vi "LSMcontroller_v64_updatedwaveformhandling.vi"() -> ()   [LabVIEW 2015] (continued)
                    n3086 = property on="wavdet" class="Bool (strict)"("Value"=FALSE ("wavdet")) -> ()  [unwired: 2 in, 2 out]
                    n3087 = local write "Save tab"(enum32{"withsave", "withoutsave"}."withsave" ("Save tab")) -> ()
                    n3088 = property on="# of frames" class="DigNum (strict)"("DisabledEnum"=T7."Enabled" ("Disabled")) -> ()  [unwired: 2 in, 2 out]
                    n3089 = property on="save\ndata" class="Bool (strict)"("DisabledEnum"=T7."Enabled" ("Disabled")) -> ()  [unwired: 2 in, 2 out]
                  }
                  frame True {
                    w6296 = FALSE ("finite samples for recording")
                    n3090 = property on="finite samples" class="Bool (strict)"("Value"=w6296) -> ()  [unwired: 2 in, 2 out]
                    n3091 = property on="wavdet" class="Bool (strict)"("Value"=w6296) -> ()  [unwired: 2 in, 2 out]
                    n3092 = property on="save\ndata" class="Bool (strict)"("Value"=w6296) -> ()  [unwired: 2 in, 2 out]
                    n3093 = local write "Save tab"(enum32{"withsave", "withoutsave"}."withsave" ("Save tab")) -> ()
                    n3094 = property on="# of frames" class="DigNum (strict)"("DisabledEnum"=T7."Disabled and Grayed Out" ("Disabled")) -> ()  [unwired: 2 in, 2 out]
                    n3095 = property on="save\ndata" class="Bool (strict)"("DisabledEnum"=T7."Disabled and Grayed Out" ("Disabled")) -> ()  [unwired: 2 in, 2 out]
                  }
                }
              }
              frame #1 {
                n3096 = local read "finite samples"() -> (w6306:bool)
                n3097 = local read "continuous"() -> (w6305:bool)
                n3098 = local read "wavdet"() -> (w6304:bool)
                n3099 = call "2pparameters.vi"("command"="get") -> ("params out"=w6300:T10)  [unwired: 1 in]
                n3100 = Bundle By Name(cluster=w6300, "finite"=w6306, "cont"=w6305, "wavdet"=w6304) -> (w6303:T10)
                n3101 = call "2pparameters.vi"("Params in"=w6303, "command"="set") -> ()  [unwired: 1 out]
              }
            }
          }
          event "wavdet": Value Change {
            n3102 = event-data() -> ("NewVal"=w6307:bool)  [unwired: 1 in]
            n3103 = flat-sequence {
              tunnel: w6307 -> [w6308]
              frame #0 {
                n3104 = case shown="False" w6308 {
                  frame False {
                    n3105 = property on="finite samples" class="Bool (strict)"("Value"=TRUE ("finite samples for recording")) -> ()  [unwired: 2 in, 2 out]
                    n3106 = property on="continuous" class="Bool (strict)"("Value"=FALSE ("continuous")) -> ()  [unwired: 2 in, 2 out]
                    n3107 = local write "Save tab"(enum32{"withsave", "withoutsave"}."withsave" ("Save tab")) -> ()
                    n3108 = property on="save\ndata" class="Bool (strict)"("DisabledEnum"=T7."Enabled" ("Disabled")) -> ()  [unwired: 2 in, 2 out]
                    n3109 = property on="# of frames" class="DigNum (strict)"("DisabledEnum"=T7."Enabled" ("Disabled")) -> ()  [unwired: 2 in, 2 out]
                    n3110 = property on="save\ndata" class="Bool (strict)"("Value"=TRUE ("save\ndata")) -> ()  [unwired: 2 in, 2 out]
                  }
                  frame True {
                    w6317 = FALSE ("finite samples for recording")
                    n3111 = property on="finite samples" class="Bool (strict)"("Value"=w6317) -> ()  [unwired: 2 in, 2 out]
                    n3112 = property on="continuous" class="Bool (strict)"("Value"=w6317) -> ()  [unwired: 2 in, 2 out]
                    n3113 = property on="save\ndata" class="Bool (strict)"("DisabledEnum"=T7."Enabled" ("Disabled")) -> ()  [unwired: 2 in, 2 out]
                    n3114 = local write "Save tab"(enum32{"withsave", "withoutsave"}."withsave" ("Save tab")) -> ()
                    n3115 = property on="# of frames" class="DigNum (strict)"("DisabledEnum"=T7."Disabled" ("Disabled")) -> ()  [unwired: 2 in, 2 out]
                    n3116 = property on="save\ndata" class="Bool (strict)"("Value"=TRUE ("save\ndata")) -> ()  [unwired: 2 in, 2 out]
                  }
                }
              }
              frame #1 {
                n3117 = local read "finite samples"() -> (w6320:bool)
                n3118 = local read "continuous"() -> (w6321:bool)
                n3119 = local read "wavdet"() -> (w6322:bool)
                n3120 = call "2pparameters.vi"("command"="get") -> ("params out"=w6326:T10)  [unwired: 1 in]
                n3121 = Bundle By Name(cluster=w6326, "finite"=w6320, "cont"=w6321, "wavdet"=w6322) -> (w6323:T10)
                n3122 = call "2pparameters.vi"("Params in"=w6323, "command"="set") -> ()  [unwired: 1 out]
              }
            }
          }
          event "cursors": Value Change {
            n3123 = event-data() -> ()  [unwired: 1 in, 5 out]
            n3124 = case shown="True" "cursors" {
              frame False {
                n3125 = property on="img_CH1" class="IntGraph (strict)"("Active Cursor"=u32 0, "Cursor.Cursor Style"=u8 0 ("Cursor Style"), "Cursor.Cursor Point Style"=u8 0 ("Cursor Point Style")) -> ("Cursor.Cursor Position:Cursor X"=w6331:dbl, "Cursor.Cursor Position:Cursor Y"=w6332:dbl)  [unwired: 2 in, 2 out]
                n3126 = property on="img_CH2" class="IntGraph (strict)"("Active Cursor"=u32 0, "Cursor.Cursor Style"=u8 0 ("Cursor Style"), "Cursor.Cursor Point Style"=u8 0 ("Cursor Point Style")) -> ()  [unwired: 2 in, 2 out]
                n3127 = local write "cursor x [pixel]"(w6331) -> ()
                n3128 = local write "cursor y [pixel]"(w6332) -> ()
              }
              frame True {
                n3129 = stacked-sequence {
                  frame #0 {
                    n3130 = call "2pparameters.vi"("command"="get") -> ("params out"=w6347:T10)  [unwired: 1 in]
                    n3131 = Unbundle By Name(w6347) -> ("Xpixels Img"=w6348:i32, "Ypixels Img"=w6345:i32)
                    n3132 = To Double Precision Float(number=w6345) -> (double precision float=w6339:dbl)
                    n3133 = To Double Precision Float(number=w6348) -> (double precision float=w6344:dbl)
                    n3134 = Divide(x=w6339, y=2.0) -> (x/y=w6340:dbl)
                    n3135 = Divide(x=w6344, y=2.0) -> (x/y=w6342:dbl)
                    n3136 = Round To Nearest(number=w6340) -> (nearest integer value=w6338:dbl)
                    n3137 = Round To Nearest(number=w6342) -> (nearest integer value=w6341:dbl)
                    n3138 = property on="img_CH1" class="IntGraph (strict)"("Active Cursor"=u32 0, "Cursor.Cursor Style"=u8 8 ("Cursor Style"), "Cursor.Cursor Point Style"=u8 5 ("Cursor Point Style"), "Cursor.Cursor Position:Cursor X"=w6341, "Cursor.Cursor Position:Cursor Y"=w6338, "Cursor.Visible"=TRUE) -> ()  [unwired: 2 in, 2 out]
                  }
                  frame #1 {
                    n3139 = call "2pparameters.vi"("command"="get") -> ("params out"=w6367:T10)  [unwired: 1 in]
                    n3140 = call "2pparameters.vi"("command"="get") -> ("params out"=w6365:T10)  [unwired: 1 in]
                    n3141 = property on="img_CH1" class="IntGraph (strict)"("Active Cursor"=u32 0, "Cursor.Cursor Style"=u8 8 ("Cursor Style"), "Cursor.Cursor Point Style"=u8 5 ("Cursor Point Style")) -> ("Cursor.Cursor Position:Cursor X"=w6360:dbl, "Cursor.Cursor Position:Cursor Y"=w6359:dbl, "Cursor.Cursor Index"=w6382:i32, "Cursor.Cursor Plot"=w6381:i32, "Cursor.Visible"=w6352:bool)  [unwired: 2 in, 2 out]
                    "cursor x [pixel]" <- w6360
                    "cursor y [pixel]" <- w6359
                    n3142 = Unbundle By Name(w6367) -> ("Vy-max Img"=w6369:dbl, "Vy-min Img"=w6356:dbl, "Ypixels Img"=w6371:i32)
                    n3143 = Unbundle By Name(w6365) -> ("VX-max Img"=w6366:dbl, "Vx-min Img"=w6354:dbl, "Xpixels Img"=w6370:i32)
                    n3144 = Subtract(x=w6369, y=w6356) -> (x-y=w6374:dbl)
                    n3145 = Subtract(x=w6366, y=w6354) -> (x-y=w6372:dbl)
                    n3146 = local read "img_CH2"() -> (w6378:sgl[][])
                    n3147 = To Double Precision Float(number=w6370) -> (double precision float=w6373:dbl)
                    n3148 = local read "img_CH1"() -> (w6379:sgl[][])
                    n3149 = To Double Precision Float(number=w6371) -> (double precision float=w6375:dbl)
                    n3150 = Index Array(array=w6379, index (row)=w6382, index (col)=w6381) -> (element=→"value CH 1":sgl)
                    n3151 = Index Array(array=w6378, index (row)=w6382, index (col)=w6381) -> (element=→"value CH 2":sgl)
                    n3152 = Divide(x=w6372, y=w6373) -> (x/y=w6376:dbl)
                    n3153 = Divide(x=w6374, y=w6375) -> (x/y=w6377:dbl)
                    n3154 = Multiply(x=w6360, y=w6376) -> (x*y=w6355:dbl)
                    n3155 = Multiply(x=w6359, y=w6377) -> (x*y=w6358:dbl)
                    n3156 = property on="img_CH2" class="IntGraph (strict)"("Active Cursor"=u32 0, "Cursor.Cursor Style"=u8 8 ("Cursor Style"), "Cursor.Cursor Point Style"=u8 5 ("Cursor Point Style"), "Cursor.Cursor Position:Cursor X"=w6360, "Cursor.Cursor Position:Cursor Y"=w6359, "Cursor.Visible"=w6352) -> ()  [unwired: 2 in, 2 out]
                    n3157 = Add(x=w6355, y=w6354) -> (x+y=w6353:dbl)
                    n3158 = Add(x=w6358, y=w6356) -> (x+y=w6357:dbl)
                    n3159 = local write "Vx-ref"(w6353) -> ()
                    n3160 = local write "Vy-ref"(w6357) -> ()
                  }
                }
              }
            }
          }
          event "img_CH1": Cursor Move {
            n3161 = event-data() -> ("CursIdx"=w6387:i32)  [unwired: 1 in]
            n3162 = Equal To 0?(x=w6387) -> (x = 0?=w6388:bool)
            n3163 = case shown="True" w6388 {
              frame False {
              }
              frame True {
                n3164 = call "2pparameters.vi"("command"="get") -> ("params out"=w6408:T10)  [unwired: 1 in]
                n3165 = call "2pparameters.vi"("command"="get") -> ("params out"=w6410:T10)  [unwired: 1 in]
                n3166 = property on="img_CH1" class="IntGraph (strict)"("Active Cursor"=u32 0, "Cursor.Cursor Style"=u8 8 ("Cursor Style"), "Cursor.Cursor Point Style"=u8 5 ("Cursor Point Style")) -> ("Cursor.Cursor Position:Cursor X"=w6397:dbl, "Cursor.Cursor Position:Cursor Y"=w6396:dbl, "Cursor.Cursor Plot"=w6416:i32, "Cursor.Cursor Index"=w6415:i32, "Cursor.Visible"=w6389:bool)  [unwired: 2 in, 2 out]
                n3167 = Unbundle By Name(w6408) -> ("Vy-max Img"=w6406:dbl, "Vy-min Img"=w6395:dbl, "Ypixels Img"=w6404:i32)
                n3168 = Unbundle By Name(w6410) -> ("VX-max Img"=w6409:dbl, "Vx-min Img"=w6390:dbl, "Xpixels Img"=w6405:i32)
                n3169 = Subtract(x=w6406, y=w6395) -> (x-y=w6401:dbl)
                n3170 = Subtract(x=w6409, y=w6390) -> (x-y=w6403:dbl)
                n3171 = local write "cursor x [pixel]"(w6397) -> ()
                n3172 = local write "cursor y [pixel]"(w6396) -> ()
                n3173 = To Double Precision Float(number=w6405) -> (double precision float=w6402:dbl)
                n3174 = To Double Precision Float(number=w6404) -> (double precision float=w6400:dbl)
                n3175 = local read "img_CH2"() -> (w6417:sgl[][])
                n3176 = local read "img_CH1"() -> (w6420:sgl[][])
                n3177 = Index Array(array=w6417, index (row)=w6416, index (col)=w6415) -> (element=w6418:sgl)
                n3178 = Index Array(array=w6420, index (row)=w6416, index (col)=w6415) -> (element=w6419:sgl)
                n3179 = Divide(x=w6403, y=w6402) -> (x/y=w6399:dbl)
                n3180 = Divide(x=w6401, y=w6400) -> (x/y=w6398:dbl)
                n3181 = local write "value CH 2"(w6418) -> ()
                n3182 = Multiply(x=w6397, y=w6399) -> (x*y=w6392:dbl)
                n3183 = local write "value CH 1"(w6419) -> ()
                n3184 = Multiply(x=w6396, y=w6398) -> (x*y=w6394:dbl)
                n3185 = Add(x=w6392, y=w6390) -> (x+y=w6391:dbl)
                n3186 = local write "Vx-ref"(w6391) -> ()
                n3187 = Add(x=w6394, y=w6395) -> (x+y=w6393:dbl)
                n3188 = property on="img_CH2" class="IntGraph (strict)"("Active Cursor"=u32 0, "Cursor.Cursor Style"=u8 8 ("Cursor Style"), "Cursor.Cursor Point Style"=u8 5 ("Cursor Point Style"), "Cursor.Cursor Position:Cursor X"=w6397, "Cursor.Cursor Position:Cursor Y"=w6396, "Cursor.Visible"=w6389) -> ()  [unwired: 2 in, 2 out]
                n3189 = local write "Vy-ref"(w6393) -> ()
              }
            }
          }
          event "img_CH2": Cursor Move {
            n3190 = event-data() -> ("CursIdx"=w6424:i32)  [unwired: 1 in]
            n3191 = Equal To 0?(x=w6424) -> (x = 0?=w6425:bool)
            n3192 = case shown="True" w6425 {
              frame False {
              }
              frame True {
                n3193 = property on="img_CH2" class="IntGraph (strict)"("Active Cursor"=u32 0, "Cursor.Cursor Style"=u8 8 ("Cursor Style"), "Cursor.Cursor Point Style"=u8 5 ("Cursor Point Style")) -> ("Cursor.Cursor Position:Cursor X"=w6433:dbl, "Cursor.Cursor Position:Cursor Y"=w6434:dbl, "Cursor.Cursor Plot"=w6453:i32, "Cursor.Cursor Index"=w6452:i32, "Cursor.Visible"=w6426:bool)  [unwired: 2 in, 2 out]
                n3194 = call "2pparameters.vi"("command"="get") -> ("params out"=w6445:T10)  [unwired: 1 in]
                n3195 = call "2pparameters.vi"("command"="get") -> ("params out"=w6447:T10)  [unwired: 1 in]
                n3196 = local read "img_CH1"() -> (w6457:sgl[][])
                n3197 = local read "img_CH2"() -> (w6454:sgl[][])
                n3198 = local write "cursor x [pixel]"(w6433) -> ()
                n3199 = local write "cursor y [pixel]"(w6434) -> ()
                n3200 = Unbundle By Name(w6445) -> ("Vy-max Img"=w6443:dbl, "Vy-min Img"=w6428:dbl, "Ypixels Img"=w6441:i32)
                n3201 = Unbundle By Name(w6447) -> ("VX-max Img"=w6446:dbl, "Vx-min Img"=w6431:dbl, "Xpixels Img"=w6442:i32)
                n3202 = Index Array(array=w6457, index (row)=w6453, index (col)=w6452) -> (element=w6456:sgl)
                n3203 = Index Array(array=w6454, index (row)=w6453, index (col)=w6452) -> (element=w6455:sgl)
                n3204 = local write "value CH 2"(w6455) -> ()
                n3205 = local write "value CH 1"(w6456) -> ()
                n3206 = Subtract(x=w6443, y=w6428) -> (x-y=w6438:dbl)
                n3207 = Subtract(x=w6446, y=w6431) -> (x-y=w6440:dbl)
                n3208 = To Double Precision Float(number=w6442) -> (double precision float=w6439:dbl)
                n3209 = To Double Precision Float(number=w6441) -> (double precision float=w6437:dbl)
                n3210 = Divide(x=w6440, y=w6439) -> (x/y=w6436:dbl)
                n3211 = Divide(x=w6438, y=w6437) -> (x/y=w6435:dbl)
                n3212 = Multiply(x=w6433, y=w6436) -> (x*y=w6432:dbl)
                n3213 = Multiply(x=w6434, y=w6435) -> (x*y=w6429:dbl)
                n3214 = property on="img_CH1" class="IntGraph (strict)"("Active Cursor"=u32 0, "Cursor.Cursor Style"=u8 8 ("Cursor Style"), "Cursor.Cursor Point Style"=u8 5 ("Cursor Point Style"), "Cursor.Cursor Position:Cursor X"=w6433, "Cursor.Cursor Position:Cursor Y"=w6434, "Cursor.Visible"=w6426) -> ()  [unwired: 2 in, 2 out]
                n3215 = Add(x=w6432, y=w6431) -> (x+y=→"Vx-ref":dbl)
                n3216 = Add(x=w6429, y=w6428) -> (x+y=→"Vy-ref":dbl)
              }
            }
          }
          event "Focus": Value Change {
            n3217 = event-data() -> ()  [unwired: 1 in, 6 out]
            n3218 = flat-sequence {
              frame #0 {
                n3219 = local read "Focus"() -> (w6461:bool)
                n3220 = case shown="True" w6461 {
                  frame False {
                  }
                  frame True {
                    n3221 = local read "Vx-ref"() -> (w6465:dbl)
                    n3222 = local read "Vy-ref"() -> (w6464:dbl)
                    n3223 = local read "zV"() -> (w6462:dbl)
                    n3224 = call "focusvi.vi"("zc"=w6462, "yc"=w6464, "xc"=w6465) -> ("finalz"=→"zV":dbl)
                  }
                }
              }
              frame #1 {
                n3225 = local write "Focus"(FALSE ("Focus")) -> ()
              }
            }
          }
          event "auto shutter": Value Change {
            n3226 = event-data() -> ()  [unwired: 1 in, 6 out]
            n3227 = call "2pparameters.vi"("command"="get") -> ("params out"=w6469:T10)  [unwired: 1 in]
            n3228 = in-place {
              n3229 = in-place-cluster #46(w6469) -> ()  [unwired: 1 out]
              n3230 = local read "auto shutter"() -> (w6471:bool)
              n3231 = in-place-cluster #46("autoshutter"=w6471) -> (w6467:T10)
            }
            n3232 = call "2pparameters.vi"("Params in"=w6467, "command"="set") -> ()  [unwired: 1 out]
          }
          event "auto OD": Value Change {
            n3233 = event-data() -> ()  [unwired: 1 in, 6 out]
            n3234 = call "2pparameters.vi"("command"="get") -> ("params out"=w6474:T10)  [unwired: 1 in]
            n3235 = in-place {
              n3236 = in-place-cluster #47(w6474) -> ()  [unwired: 1 out]
              n3237 = local read "auto OD"() -> (w6476:bool)
              n3238 = in-place-cluster #47("auto OD"=w6476) -> (w6472:T10)
            }
            n3239 = call "2pparameters.vi"("Params in"=w6472, "command"="set") -> ()  [unwired: 1 out]
          }
          event "ODfilt": Value Change {
            n3240 = event-data() -> ("OldVal"=w6477:u16)  [unwired: 1 in, 5 out]
            n3241 = local read "ODfilt"() -> (w6478:u16)
            n3242 = call "2pparameters.vi"("command"="get") -> ("params out"=w6481:T10)  [unwired: 1 in]
            n3243 = call "filterwheelcontrol_nothorlabslib.vi"("Current OD filt"=w6477, "New ODfilt"=w6478) -> ()  [unwired: 1 in]
            n3244 = in-place {
              in-place-border: w6478 -> [w6483]
              n3245 = in-place-cluster #48(w6481) -> ()  [unwired: 1 out]
              n3246 = in-place-cluster #48("ODfilt"=w6483) -> (w6479:T10)
            }
            n3247 = call "2pparameters.vi"("Params in"=w6479, "command"="set") -> ()  [unwired: 1 out]
          }
          event "Exit": Value Change {
            n3248 = event-data() -> ()  [unwired: 1 in, 5 out]
          }
        }
        n3249 = Wait (ms)(milliseconds to wait=u32 50) -> ()  [unwired: 1 out]
      }
      n3250 = while {
        stop <- w69 stop-if-true
        # "Waveform generation"
        n3251 = event shown="[15] \"Update settings\": Value Change" {
          selector: _ -> [_ _ _ _ _ _ _ _ _ _ _ _ _ _ _ _ _ _ _ _ _ _]
          dyn-events: _ -> [_ _ _ _ _ _ _ _ _ _ _ _ _ _ _ _ _ _ _ _ _ _]
          timeout: _ -> [_ _ _ _ _ _ _ _ _ _ _ _ _ _ _ _ _ _ _ _ _ _]
          tunnel: [_ _ _ _ _ _ _ _ _ _ _ _ _ _ _ _ _ _ _ _ _ w2081] -> w69
          event Timeout {
            n3252 = event-data() -> ()  [unwired: 1 in, 3 out]
          }
          event "Add AO wave": Value Change {
            n3253 = event-data() -> ("NewVal"=w70:bool)  [unwired: 1 in, 5 out]
            n3254 = case shown="True" w70 {
              frame False {
              }
              frame True {
                n3255 = stacked-sequence {
                  frame #0 {
                    n3256 = local read "Measurement"() -> (w71:T4)
                    n3257 = case shown="\"Lifetime (contour)\"" w71 {
                      frame "X-Y-t movie", Default {
                        n3258 = local read "avpp"() -> (w92:i32)
                        n3259 = local read "Angle ref"() -> (w91:dbl)
                        n3260 = local read "ROI Type"() -> (w90:u16)
                        n3261 = local read "xpixels ref"() -> (w87:i32)
                        n3262 = local read "Vx-min ref"() -> (w86:dbl)
                        n3263 = local read "Vx-max ref"() -> (w85:dbl)
                        n3264 = local read "ypixels ref"() -> (w83:i32)
                        n3265 = local read "Vy-min ref"() -> (w84:dbl)
                        n3266 = local read "Vy-max ref"() -> (w80:dbl)
                        n3267 = local read "Sampling rate"() -> (w74:dbl)
                        n3268 = local read "finite samples"() -> (w75:bool)
                        n3269 = local read "continuous"() -> (w78:bool)
                        n3270 = local read "wavdet"() -> (w79:bool)
                        n3271 = local read "# of frames"() -> (w77:i32)
                        n3272 = local read "maxbufferAI"() -> (w76:i32)
                        n3273 = local read "Override AI buffer"() -> (w72:bool)
                        n3274 = call "2pparameters.vi"("command"="get") -> ("params out"=w89:T10)  [unwired: 1 in]
                        n3275 = Bundle By Name(cluster=w89, "type"="X-Y-t movie", "avpp"=w92, "Angle Img"=w91, "Xpixels Img"=w87, "Vx-min Img"=w86, "VX-max Img"=w85, "Ypixels Img"=w83, "Vy-min Img"=w84, "Vy-max Img"=w80, "srate"=w74, "srate Img"=w74, "finite"=w75, "cont"=w78, "wavdet"=w79, "measpoints"=w77, "maxbufferAI"=w76, "Drawing Mode"=w90, "Vz-reset"=0.0, "AIoverride"=w72) -> (w81:T10)
                        n3276 = call "2pparameters.vi"("Params in"=w81, "command"="set") -> ()  [unwired: 1 out]
                      }
                      frame "X-Y-Z stack" {
                        n3277 = call "2pparameters.vi"("command"="get") -> ("params out"=w96:T10)  [unwired: 1 in]
                        n3278 = Bundle By Name(cluster=w96, "type"="X-Y-Z stack") -> (w94:T10)
                        n3279 = call "2pparameters.vi"("Params in"=w94, "command"="set") -> ()  [unwired: 1 out]
                      }
                      frame "Lifetime (scan)" {
                        n3280 = call "2pparameters.vi"("command"="get") -> ("params out"=w101:T10)  [unwired: 1 in]
                        n3281 = Bundle By Name(cluster=w101, "type"="Lifetime (scan)") -> (w99:T10)
                        n3282 = call "2pparameters.vi"("Params in"=w99, "command"="set") -> ()  [unwired: 1 out]
                      }
                      frame "Lifetime (contour)" {
                        n3283 = local read "Vy-min draw"() -> (w111:dbl)
                        n3284 = local read "Vy-max draw"() -> (w110:dbl)
                        n3285 = local read "Vx-min draw"() -> (w113:dbl)
                        n3286 = local read "Vx-max draw"() -> (w112:dbl)
                        n3287 = local read "xpixels ref"() -> (w109:i32)
                        n3288 = local read "ypixels ref"() -> (w108:i32)
                        n3289 = local read "ROI Type"() -> (w107:u16)
                        n3290 = local read "srateAODOtt"() -> (w118:dbl)
                        n3291 = local read "# of frames"() -> (w123:i32)
                        n3292 = local read "refreshtime"() -> (w115:dbl)
                        n3293 = local read "Pel"() -> (w106:dbl)
                        n3294 = local read "bin"() -> (w121:dbl)
                        n3295 = local read "Override AI buffer"() -> (w104:bool)
                        n3296 = local read "finite samples"() -> (w130:bool)
                        n3297 = local read "srateAODOtt"() -> (w117:dbl)
                        n3298 = local read "srateAODOtt"() -> (w124:dbl)
                        n3299 = local read "continuous"() -> (w129:bool)
                        n3300 = local read "Angle ref"() -> (w114:dbl)
                        n3301 = local read "wavdet"() -> (w131:bool)
                        n3302 = local read "Vx-ref"() -> (w126:dbl)
                        n3303 = local read "Vy-ref"() -> (w128:dbl)
                        n3304 = local read "avpp"() -> (w127:i32)
                        n3305 = call "tt_timeandsamples.vi"("bin"=w121, "refreshtime"=w115, "srateAODOtt"=w118, "tot#ofsamples"=w123) -> ("refreshrate"=w119:dbl, "refreshbuffer"=w120:i32, "timetracecycles"=w125:i32)  [unwired: 5 in]
                        n3306 = local read "bin"() -> (w122:dbl)
                        n3307 = call "2pparameters.vi"("command"="get") -> ("params out"=w134:T10)  [unwired: 1 in]
                        n3308 = Bundle By Name(cluster=w134, "Drawing Mode"=w107, "measpoints"=w123, "tt_cycles"=w125, "refreshbuffer"=w120, "refreshrate"=w119, "Vx-ref"=w126, "Vy-ref"=w128, "srate"=w117, "finite"=w130, "cont"=w129, "wavdet"=w131, "avpp"=w127, "srateAODO"=w124, "bufferAI"=w120, "bin"=w122, "Angle Img"=w114, "Vxminref"=w113, "Vxmaxref"=w112, "Vyminref"=w111, "Vymaxref"=w110, "Xpixels Img"=w109, "Ypixels Img"=w108, "Pel"=w106, "Vz-reset"=0.0, "AIoverride"=w104, "type"="Lifetime (contour)") -> (w132:T10)
                        n3309 = Reciprocal(x=w119) -> (1/x=w116:dbl)
                        n3310 = local write "refreshtime"(w116) -> ()
                        n3311 = call "2pparameters.vi"("Params in"=w132, "command"="set") -> ()  [unwired: 1 out]
                      }
                      frame "X-Y-Z-t movie" {
                      }
                      frame "linescan" {
                      }
                      frame "Timetrace" {
                        n3312 = local read "Vy-min draw"() -> (w144:dbl)
                        n3313 = local read "Vy-max draw"() -> (w143:dbl)
                        n3314 = local read "Vx-min draw"() -> (w146:dbl)
                        n3315 = local read "Vx-max draw"() -> (w145:dbl)
                        n3316 = local read "xpixels ref"() -> (w142:i32)
                        n3317 = local read "ypixels ref"() -> (w141:i32)
                        n3318 = local read "ROI Type"() -> (w140:u16)
                        n3319 = local read "srateAODOtt"() -> (w151:dbl)
                        n3320 = local read "# of frames"() -> (w156:i32)
                        n3321 = local read "refreshtime"() -> (w148:dbl)
                        n3322 = local read "Pel"() -> (w139:dbl)
                        n3323 = local read "bin"() -> (w154:dbl)
                        n3324 = local read "Override AI buffer"() -> (w137:bool)
                        n3325 = local read "finite samples"() -> (w163:bool)
                        n3326 = local read "srateAODOtt"() -> (w150:dbl)
                        n3327 = local read "srateAODOtt"() -> (w157:dbl)
                        n3328 = local read "continuous"() -> (w162:bool)
                        n3329 = local read "Angle ref"() -> (w147:dbl)
                        n3330 = local read "wavdet"() -> (w164:bool)
                        n3331 = local read "Vx-ref"() -> (w159:dbl)
                        n3332 = local read "Vy-ref"() -> (w161:dbl)
                        n3333 = local read "avpp"() -> (w160:i32)
                        n3334 = call "tt_timeandsamples.vi"("bin"=w154, "refreshtime"=w148, "srateAODOtt"=w151, "tot#ofsamples"=w156) -> ("refreshrate"=w152:dbl, "refreshbuffer"=w153:i32, "timetracecycles"=w158:i32)  [unwired: 5 in]
                        n3335 = local read "bin"() -> (w155:dbl)
                        n3336 = call "2pparameters.vi"("command"="get") -> ("params out"=w167:T10)  [unwired: 1 in]
                        n3337 = Bundle By Name(cluster=w167, "Drawing Mode"=w140, "measpoints"=w156, "tt_cycles"=w158, "refreshbuffer"=w153, "refreshrate"=w152, "Vx-ref"=w159, "Vy-ref"=w161, "srate"=w150, "finite"=w163, "cont"=w162, "wavdet"=w164, "avpp"=w160, "srateAODO"=w157, "bufferAI"=w153, "bin"=w155, "Angle Img"=w147, "Vxminref"=w146, "Vxmaxref"=w145, "Vyminref"=w144, "Vymaxref"=w143, "Xpixels Img"=w142, "Ypixels Img"=w141, "Pel"=w139, "Vz-reset"=0.0, "AIoverride"=w137, "type"="Timetrace") -> (w165:T10)
                        n3338 = Reciprocal(x=w152) -> (1/x=w149:dbl)
                        n3339 = local write "refreshtime"(w149) -> ()
                        n3340 = call "2pparameters.vi"("Params in"=w165, "command"="set") -> ()  [unwired: 1 out]
                      }
                      frame "Lifetime (point)" {
                      }
                    }
                  }
                  frame #1 {
                    w170 = FALSE ("wavdet")
                    n3341 = call "2pparameters.vi"("command"="get") -> ("params out"=w174:T10)  [unwired: 1 in]
                    n3342 = Bundle By Name(cluster=w174, "finite"=w170, "cont"=w170, "wavdet"=TRUE) -> (w171:T10)
                    n3343 = call "2pparameters.vi"("Params in"=w171, "command"="set") -> ()  [unwired: 1 out]
                  }
                  frame #2 {
                    # "change active waveform numbers array"
                    n3344 = local read "AO channels"() -> (w181:u32)
                    n3345 = call "2pparameters.vi"("command"="get") -> ("params out"=w179:T10)  [unwired: 1 in]
                    n3346 = in-place {
                      in-place-border: w181 -> [w185]
                      in-place-border: [w182] -> w176
                      n3347 = in-place-cluster #49(w179) -> ("aAO"=w184:u32[])
                      n3348 = call "add channel to active arrayv2.vi"("line array in"=w184, "line to add"=w185) -> ("line array out"=w183:u32[], "addition"=w182:bool)  [unwired: 1 out]
                      n3349 = in-place-cluster #49("aAO"=w183) -> (w177:T10)
                    }
                    n3350 = local write "addAO"(w176) -> ()
                    n3351 = call "2pparameters.vi"("Params in"=w177, "command"="set") -> ()  [unwired: 1 out]
                  }
                  frame #3 {
                    # "update GUI"
                    n3352 = local read "addAO"() -> (w186:bool)
                    n3353 = case shown="True" w186 {
                      frame False {
                      }
                      frame True {
                        n3354 = call "Used AO lines.vi"() -> ("used AO names"=w190:string[], "used AO lines"=w192:tag[])  [unwired: 2 in]
                        n3355 = control-ref of="Analog Lines Plot"() -> (w191:refnum<vi>)
                        n3356 = control-ref of="Digital Lines Plot"() -> (w189:refnum<vi>)
                        n3357 = call "Used DO lines.vi"() -> ("used DO names"=w188:string[], "used DO lines"=w187:tag[])  [unwired: 2 in]
                        n3358 = local write "Analog Used Lines"(w192) -> ()
                        n3359 = local write "Analog Used Names"(w190) -> ()
                        n3360 = local write "Digital Used Lines"(w187) -> ()
                        n3361 = local write "Digital Used Names"(w188) -> ()
                        n3362 = call "prepDOWaveplot.vi"("DigitalGraph in"=w189, "used DO names"=w188) -> ()  [unwired: 1 in]
                        n3363 = call "prepAOWaveplot.vi"("WaveformGraph in"=w191, "Analog Used Names"=w190) -> ()  [unwired: 1 in]
                      }
                    }
                  }
                  frame #4 {
                    n3364 = local read "addAO"() -> (w193:bool)
                    n3365 = case shown="True" w193 {
                      frame False {
                      }
                      frame True {
                        # "add parameters\nto parameter array"
                        n3366 = local read "Build analog waveform tabs"() -> (w194:enum32{"Square", "Triangle", "Matlab"})
                        n3367 = case shown="\"Matlab\"" w194 {
                          frame "Square", Default {
                            w207 = 0.0 ("Offset (V)")
                            n3368 = local read "Meastab"() -> (w196:enum32{"X-Y Image", "Linescan", "Timetrace"})
                            n3369 = call "waveformparamsv2.vi"("command"="get") -> ("Params out"=w205:T14)  [unwired: 4 in, 2 out]
                            n3370 = Unbundle By Name(w205) -> ("AO parameters"=w202:T15)
                            n3371 = case shown="\"Timetrace\"" w196 {
                              tunnel: [w218 w219] -> w195
                              frame "X-Y Image", Default {
                                n3372 = local read "Sampling rate"() -> (w218:dbl)
                              }
                              frame "Timetrace" {
                                n3373 = local read "srateAODOtt"() -> (w219:dbl)
                              }
                            }
                            n3374 = local read "Start amplitude (V)"() -> (w215:dbl)
                            n3375 = local read "phase shift (ms)"() -> (w208:dbl)
                            n3376 = local read "Step size (V)"() -> (w213:dbl)
                            n3377 = local read "Baseline (V)"() -> (w214:dbl)
                            n3378 = local read "Period (ms)"() -> (w211:dbl)
                            n3379 = local read "padding value"() -> (w198:dbl)
                            n3380 = local read "Repeats"() -> (w217:dbl)
                            n3381 = local read "DC (%)"() -> (w212:dbl)
                            n3382 = local read "Cycles"() -> (w216:dbl)
                            n3383 = local read "Pulses"() -> (w209:dbl)
                            n3384 = Index Array(array=w202, index=0) -> (element=w203:T16)
                            n3385 = Bundle By Name(cluster=w203, "AOtab"=0.0 ("Repeats"), "Repeats"=w217, "Cycles"=w216, "Start amplitude (V)"=w215, "Baseline (V)"=w214, "Step size (V)"=w213, "DC (%)"=w212, "Sampling frequency (Hz)"=w195, "Period (ms)"=w211, "Offset (V)"=w207, "Amplitude (V)"=w207, "Frequency"=w207, "Tri Repeats"=w207, "phase shift (ms)"=w208, "Pulses"=w209, "Matlab wave file"=path "", "padding value"=w198) -> (w200:T16)
                            n3386 = Build Array(w200) -> (w199:T15)
                            n3387 = call "waveformparamsv2.vi"("command"="add AO", "add AO"=w199) -> ()  [unwired: 3 in, 3 out]
                          }
                          frame "Matlab" {
                            w225 = 0.0 ("Repeats")
                            n3388 = local read "Meastab"() -> (w221:enum32{"X-Y Image", "Linescan", "Timetrace"})
                            n3389 = call "waveformparamsv2.vi"("command"="get") -> ("Params out"=w232:T14)  [unwired: 4 in, 2 out]
                            n3390 = Unbundle By Name(w232) -> ("AO parameters"=w229:T15)
                            n3391 = case shown="\"Timetrace\"" w221 {
                              tunnel: [w235 w236] -> w220
                              frame "X-Y Image", Default {
                                n3392 = local read "Sampling rate"() -> (w235:dbl)
                              }
                              frame "Timetrace" {
                                n3393 = local read "srateAODOtt"() -> (w236:dbl)
                              }
                            }
                            n3394 = local read "Matlab waveform path"() -> (w222:path)
                            n3395 = local read "Matlab padding value"() -> (w224:dbl)
                            n3396 = Index Array(array=w229, index=0) -> (element=w230:T16)
                            n3397 = call "matlabwfexistsdialogue.vi"("Matlab waveform path"=w222) -> ("mtalab waveform path out"=w223:path)
                            n3398 = Bundle By Name(cluster=w230, "AOtab"=2.0 ("Repeats"), "Repeats"=w225, "Cycles"=w225, "Start amplitude (V)"=w225, "Baseline (V)"=w225, "Step size (V)"=w225, "DC (%)"=w225, "Sampling frequency (Hz)"=w220, "Period (ms)"=w225, "Offset (V)"=w225, "Amplitude (V)"=w225, "Frequency"=w225, "Tri Repeats"=w225, "phase shift (ms)"=w225, "Pulses"=w225, "Matlab wave file"=w223, "padding value"=w224) -> (w227:T16)
                            n3399 = Build Array(w227) -> (w226:T15)
                            n3400 = call "waveformparamsv2.vi"("command"="add AO", "add AO"=w226) -> ()  [unwired: 3 in, 3 out]
                          }
                          frame "Triangle" {
                            w242 = 0.0 ("Offset (V)")
                            n3401 = local read "Meastab"() -> (w238:enum32{"X-Y Image", "Linescan", "Timetrace"})
                            n3402 = call "waveformparamsv2.vi"("command"="get") -> ("Params out"=w254:T14)  [unwired: 4 in, 2 out]
                            n3403 = Unbundle By Name(w254) -> ("AO parameters"=w251:T15)
                            n3404 = case shown="\"Timetrace\"" w238 {
                              tunnel: [w256 w257] -> w237
                              frame "X-Y Image", Default {
                                n3405 = local read "Sampling rate"() -> (w256:dbl)
                              }
                              frame "Timetrace" {
                                n3406 = local read "srateAODOtt"() -> (w257:dbl)
                              }
                            }
                            n3407 = local read "Tri padding value"() -> (w240:dbl)
                            n3408 = local read "Amplitude (V)"() -> (w245:dbl)
                            n3409 = local read "Tri Phase (s)"() -> (w241:dbl)
                            n3410 = local read "Tri Repeats"() -> (w243:dbl)
                            n3411 = local read "Frequency"() -> (w244:dbl)
                            n3412 = local read "Offset (V)"() -> (w246:dbl)
                            n3413 = Index Array(array=w251, index=0) -> (element=w252:T16)
                            n3414 = Bundle By Name(cluster=w252, "AOtab"=1.0 ("Repeats"), "Repeats"=w242, "Cycles"=w242, "Start amplitude (V)"=w242, "Baseline (V)"=w242, "Step size (V)"=w242, "DC (%)"=w242, "Sampling frequency (Hz)"=w237, "Period (ms)"=w242, "Offset (V)"=w246, "Amplitude (V)"=w245, "Frequency"=w244, "Tri Repeats"=w243, "phase shift (ms)"=w242, "Pulses"=w242, "Matlab wave file"=path "", "Tri phase"=w241, "padding value"=w240) -> (w249:T16)
                            n3415 = Build Array(w249) -> (w248:T15)
                            n3416 = call "waveformparamsv2.vi"("command"="add AO", "add AO"=w248) -> ()  [unwired: 3 in, 3 out]
                          }
                        }
                      }
                    }
                  }
                  frame #5 {
                    n3417 = local read "addAO"() -> (w258:bool)
                    n3418 = case shown="True" w258 {
                      frame False {
                      }
                      frame True {
                        # "add waveform to waveform array; correct waveform lengths and plot"
                        n3419 = local read "Meastab"() -> (w262:enum32{"X-Y Image", "Linescan", "Timetrace"})
                        n3420 = local read "Build analog waveform tabs"() -> (w272:enum32{"Square", "Triangle", "Matlab"})
                        n3421 = case shown="\"Timetrace\"" w262 {
                          tunnel: [w280 w281] -> w261
                          frame "X-Y Image", Default {
                            n3422 = local read "Sampling rate"() -> (w280:dbl)
                          }
                          frame "Timetrace" {
                            n3423 = local read "srateAODOtt"() -> (w281:dbl)
                          }
                        }
                        n3424 = call "waveformparamsv2.vi"("command"="get last AO") -> ("last AO"=w274:T16)  [unwired: 4 in, 2 out]
                        n3425 = case shown="\"Matlab\"" w272 {
                          tunnel: w274 -> [w284 w286 w288]
                          tunnel: [w283 w285 w287] -> w273
                          frame "Square", Default {
                            n3426 = call "generateRampedSquareWave_fromAOparameters.vi"("AO params"=w284) -> ("Waveform"=w283:waveform(dbl))  [unwired: 1 out]
                          }
                          frame "Triangle" {
                            n3427 = call "generateTriWave_fromAOparameters.vi"("AO params"=w286) -> ("Waveform"=w285:waveform(dbl))  [unwired: 1 out]
                          }
                          frame "Matlab" {
                            n3428 = call "matlabAOwffromparam.vi"("Cluster"=w288) -> ("Waveform"=w287:waveform(dbl))  [unwired: 1 out]
                          }
                        }
                        n3429 = property on="refwf" class="Ring (strict)"() -> ("RingText.Text"=w265:string)  [unwired: 2 in, 2 out]
                        n3430 = call "waveformsAObuffer.vi"("command"="get") -> ("AO wf out"=w278:waveform(dbl)[])  [unwired: 1 in]
                        n3431 = Build Array (concatenate)(w278, w273) -> (w275:waveform(dbl)[])
                        n3432 = call "waveformsDObuffer.vi"("command"="get") -> ("DO wf out"=w270:digitalwaveform[])  [unwired: 1 in]
                        n3433 = call "correctwaveformsizetemp.vi"("new sampling frequency (Hz)"=w261, "start"=FALSE, "reference waveforms to"=w265, "Analog waveforms in"=w275, "stop"=FALSE, "Digital waveforms in"=w270) -> ("analog wf out"=w268:waveform(dbl)[], "Digital wf out"=w266:digitalwaveform[], "measpoints"=w263:i32)
                        n3434 = local write "Analog Lines Plot"(w268) -> ()
                        n3435 = call "GetNumCamFramesv2.vi"("Digital Waveform Graph"=w266) -> ("Numeric"=w267:i32)  [unwired: 10 in]
                        n3436 = local write "Digital Lines Plot"(w266) -> ()
                        n3437 = call "waveformsAObuffer.vi"("AO wf in"=w268, "command"="set") -> ()  [unwired: 1 out]
                        n3438 = call "waveformsDObuffer.vi"("DO wf in"=w266, "command"="set") -> ()  [unwired: 1 out]
                        n3439 = local write "Total Camera Frames"(w267) -> ()
                        n3440 = local read "wavdet"() -> (w264:bool)
                        n3441 = case shown="True" w264 {
                          tunnel: w263 -> [_ w282]
                          frame False {
                          }
                          frame True {
                            n3442 = local write "# of frames"(w282) -> ()
                          }
                        }
                      }
                    }
                  }
                  frame #6 {
                    w290 = FALSE ("addAO")
                    # "set signaling boolean to false"
                    n3443 = local read "Build analog waveform tabs"() -> (w289:enum32{"Square", "Triangle", "Matlab"})
                    n3444 = local read "finite samples"() -> (w291:bool)
                    n3445 = local read "continuous"() -> (w292:bool)
                    n3446 = local read "wavdet"() -> (w293:bool)
                    n3447 = call "2pparameters.vi"("command"="get") -> ("params out"=w296:T10)  [unwired: 1 in]
                    n3448 = Bundle By Name(cluster=w296, "finite"=w291, "cont"=w292, "wavdet"=w293) -> (w294:T10)
                    n3449 = case shown="\"Matlab\"" w289 {
                      frame "Square", Default {
                        n3450 = local write "not loaded"(FALSE ("not loaded")) -> ()
                      }
                      frame "Triangle" {
                        n3451 = local write "not loadedtri"(FALSE ("not loadedtri")) -> ()
                      }
                      frame "Matlab" {
                        n3452 = local write "not loadedml"(FALSE ("not loadedml")) -> ()
                      }
                    }
                    n3453 = local write "addAO"(w290) -> ()
                    n3454 = property on="Add AO wave" class="Bool (strict)"("Val(Sgnl)"=w290) -> ()  [unwired: 2 in, 2 out]
                    n3455 = call "2pparameters.vi"("Params in"=w294, "command"="set") -> ()  [unwired: 1 out]
                  }
                }
              }
            }
          }
          event "AO channels": Value Change {
            n3456 = event-data() -> ()  [unwired: 1 in, 6 out]
            n3457 = local read "AO channels"() -> (w301:u32)
            n3458 = call "2pparameters.vi"("command"="get") -> ("params out"=w303:T10)  [unwired: 1 in]
            n3459 = Unbundle By Name(w303) -> ("aAO"=w302:u32[])
            n3460 = Search 1D Array(1D array=w302, element=w301) -> (index of element=w305:i32)  [unwired: 1 in]
            n3461 = Equal?(x=w305, y=-1.0) -> (x = y?=w306:bool)
            n3462 = case shown="False" w306 {
              tunnel: w305 -> [w308 _]
              frame False {
                n3463 = call "waveformparamsv2.vi"("command"="get") -> ("Params out"=w315:T14)  [unwired: 4 in, 2 out]
                n3464 = Unbundle By Name(w315) -> ("AO parameters"=w314:T15)
                n3465 = Index Array(array=w314, index=w308) -> (element=w331:T16)
                n3466 = Unbundle By Name(w331) -> ("AOtab"=w312:dbl, "Repeats"=w330:dbl, "Cycles"=w329:dbl, "Start amplitude (V)"=w328:dbl, "Baseline (V)"=w327:dbl, "Step size (V)"=w326:dbl, "DC (%)"=w325:dbl, "Sampling frequency (Hz)"=w324:dbl, "Period (ms)"=w323:dbl, "Offset (V)"=w322:dbl, "Amplitude (V)"=w321:dbl, "Frequency"=w320:dbl, "Tri Repeats"=w319:dbl, "phase shift (ms)"=w318:dbl, "Pulses"=w317:dbl, "Tri phase"=w313:dbl, "padding value"=w309:dbl, "Matlab wave file"=w310:path)
                n3467 = To Unsigned Long Integer(number=w312) -> (unsigned 32bit integer=w311:u32)
                n3468 = local write "Build analog waveform tabs"(w311) -> ()
                n3469 = local write "Matlab waveform path"(w310) -> ()
                n3470 = local write "phase shift (ms)"(w318) -> ()
                n3471 = local write "Repeats"(w330) -> ()
                n3472 = local write "Cycles"(w329) -> ()
                n3473 = local write "Amplitude (V)"(w321) -> ()
                n3474 = local write "Matlab padding value"(w309) -> ()
                n3475 = local write "Tri padding value"(w309) -> ()
                n3476 = local write "Start amplitude (V)"(w328) -> ()
                n3477 = local write "Tri Phase (s)"(w313) -> ()
                n3478 = local write "Period (ms)"(w323) -> ()
                n3479 = local write "Tri Repeats"(w319) -> ()
                n3480 = local write "Offset (V)"(w322) -> ()
                n3481 = local write "Frequency"(w320) -> ()
                n3482 = local write "Pulses"(w317) -> ()
                n3483 = local write "padding value"(w309) -> ()
                n3484 = local write "Sampling rate \ncurrent wf"(w324) -> ()
                n3485 = local write "Baseline (V)"(w327) -> ()
                n3486 = local write "Step size (V)"(w326) -> ()
                n3487 = local write "DC (%)"(w325) -> ()
              }
              frame True {
              }
            }
          }
          event "Rem AO wave": Value Change {
            n3488 = event-data() -> ("NewVal"=w332:bool)  [unwired: 1 in, 5 out]
            n3489 = case shown="True" w332 {
              frame False {
              }
              frame True {
                n3490 = stacked-sequence {
                  seq-local: [_ _ w438 _ _ _ _] -> [_ _ _ _ w458 w461 _]
                  frame #0 {
                    n3491 = local read "Measurement"() -> (w333:T4)
                    n3492 = case shown="\"X-Y-t movie\", Default" w333 {
                      frame "X-Y-t movie", Default {
                        n3493 = local read "avpp"() -> (w354:i32)
                        n3494 = local read "Angle ref"() -> (w353:dbl)
                        n3495 = local read "ROI Type"() -> (w352:u16)
                        n3496 = local read "xpixels ref"() -> (w349:i32)
                        n3497 = local read "Vx-min ref"() -> (w348:dbl)
                        n3498 = local read "Vx-max ref"() -> (w347:dbl)
                        n3499 = local read "ypixels ref"() -> (w345:i32)
                        n3500 = local read "Vy-min ref"() -> (w346:dbl)
                        n3501 = local read "Vy-max ref"() -> (w342:dbl)
                        n3502 = local read "Sampling rate"() -> (w336:dbl)
                        n3503 = local read "finite samples"() -> (w337:bool)
                        n3504 = local read "continuous"() -> (w340:bool)
                        n3505 = local read "wavdet"() -> (w341:bool)
                        n3506 = local read "# of frames"() -> (w339:i32)
                        n3507 = local read "maxbufferAI"() -> (w338:i32)
                        n3508 = local read "Override AI buffer"() -> (w334:bool)
                        n3509 = call "2pparameters.vi"("command"="get") -> ("params out"=w351:T10)  [unwired: 1 in]
                        n3510 = Bundle By Name(cluster=w351, "type"="X-Y-t movie", "avpp"=w354, "Angle Img"=w353, "Xpixels Img"=w349, "Vx-min Img"=w348, "VX-max Img"=w347, "Ypixels Img"=w345, "Vy-min Img"=w346, "Vy-max Img"=w342, "srate"=w336, "srate Img"=w336, "finite"=w337, "cont"=w340, "wavdet"=w341, "measpoints"=w339, "maxbufferAI"=w338, "Drawing Mode"=w352, "Vz-reset"=0.0, "AIoverride"=w334) -> (w343:T10)
                        n3511 = call "2pparameters.vi"("Params in"=w343, "command"="set") -> ()  [unwired: 1 out]
                      }
                      frame "X-Y-Z stack" {
                        n3512 = call "2pparameters.vi"("command"="get") -> ("params out"=w358:T10)  [unwired: 1 in]
                        n3513 = Bundle By Name(cluster=w358, "type"="X-Y-Z stack") -> (w356:T10)
                        n3514 = call "2pparameters.vi"("Params in"=w356, "command"="set") -> ()  [unwired: 1 out]
                      }
                      frame "Lifetime (scan)" {
                        n3515 = call "2pparameters.vi"("command"="get") -> ("params out"=w363:T10)  [unwired: 1 in]
                        n3516 = Bundle By Name(cluster=w363, "type"="Lifetime (scan)") -> (w361:T10)
                        n3517 = call "2pparameters.vi"("Params in"=w361, "command"="set") -> ()  [unwired: 1 out]
                      }
                      frame "Lifetime (contour)" {
                        n3518 = local read "Vy-min draw"() -> (w373:dbl)
                        n3519 = local read "Vy-max draw"() -> (w372:dbl)
                        n3520 = local read "Vx-min draw"() -> (w375:dbl)
                        n3521 = local read "Vx-max draw"() -> (w374:dbl)
                        n3522 = local read "xpixels ref"() -> (w371:i32)
                        n3523 = local read "ypixels ref"() -> (w370:i32)
                        n3524 = local read "ROI Type"() -> (w369:u16)
                        n3525 = local read "srateAODOtt"() -> (w380:dbl)
                        n3526 = local read "# of frames"() -> (w385:i32)
                        n3527 = local read "refreshtime"() -> (w377:dbl)
                        n3528 = local read "Pel"() -> (w368:dbl)
                        n3529 = local read "bin"() -> (w383:dbl)
                        n3530 = local read "Override AI buffer"() -> (w366:bool)
                        n3531 = local read "finite samples"() -> (w392:bool)
                        n3532 = local read "srateAODOtt"() -> (w379:dbl)
                        n3533 = local read "srateAODOtt"() -> (w386:dbl)
                        n3534 = local read "continuous"() -> (w391:bool)
                        n3535 = local read "Angle ref"() -> (w376:dbl)
                        n3536 = local read "wavdet"() -> (w393:bool)
                        n3537 = local read "Vx-ref"() -> (w388:dbl)
                        n3538 = local read "Vy-ref"() -> (w390:dbl)
                        n3539 = local read "avpp"() -> (w389:i32)
                        n3540 = call "tt_timeandsamples.vi"("bin"=w383, "refreshtime"=w377, "srateAODOtt"=w380, "tot#ofsamples"=w385) -> ("refreshrate"=w381:dbl, "refreshbuffer"=w382:i32, "timetracecycles"=w387:i32)  [unwired: 5 in]
                        n3541 = local read "bin"() -> (w384:dbl)
                        n3542 = call "2pparameters.vi"("command"="get") -> ("params out"=w396:T10)  [unwired: 1 in]
                        n3543 = Bundle By Name(cluster=w396, "Drawing Mode"=w369, "measpoints"=w385, "tt_cycles"=w387, "refreshbuffer"=w382, "refreshrate"=w381, "Vx-ref"=w388, "Vy-ref"=w390, "srate"=w379, "finite"=w392, "cont"=w391, "wavdet"=w393, "avpp"=w389, "srateAODO"=w386, "bufferAI"=w382, "bin"=w384, "Angle Img"=w376, "Vxminref"=w375, "Vxmaxref"=w374, "Vyminref"=w373, "Vymaxref"=w372, "Xpixels Img"=w371, "Ypixels Img"=w370, "Pel"=w368, "Vz-reset"=0.0, "AIoverride"=w366, "type"="Lifetime (contour)") -> (w394:T10)
                        n3544 = Reciprocal(x=w381) -> (1/x=w378:dbl)
                        n3545 = local write "refreshtime"(w378) -> ()
                        n3546 = call "2pparameters.vi"("Params in"=w394, "command"="set") -> ()  [unwired: 1 out]
                      }
                      frame "X-Y-Z-t movie" {
                      }
                      frame "linescan" {
                      }
                      frame "Timetrace" {
                        n3547 = local read "Vy-min draw"() -> (w406:dbl)
                        n3548 = local read "Vy-max draw"() -> (w405:dbl)
                        n3549 = local read "Vx-min draw"() -> (w408:dbl)
                        n3550 = local read "Vx-max draw"() -> (w407:dbl)
                        n3551 = local read "xpixels ref"() -> (w404:i32)
                        n3552 = local read "ypixels ref"() -> (w403:i32)
                        n3553 = local read "ROI Type"() -> (w402:u16)
                        n3554 = local read "srateAODOtt"() -> (w413:dbl)
                        n3555 = local read "# of frames"() -> (w418:i32)
                        n3556 = local read "refreshtime"() -> (w410:dbl)
                        n3557 = local read "Pel"() -> (w401:dbl)
                        n3558 = local read "bin"() -> (w416:dbl)
                        n3559 = local read "Override AI buffer"() -> (w399:bool)
                        n3560 = local read "finite samples"() -> (w425:bool)
                        n3561 = local read "srateAODOtt"() -> (w412:dbl)
                        n3562 = local read "srateAODOtt"() -> (w419:dbl)
                        n3563 = local read "continuous"() -> (w424:bool)
                        n3564 = local read "Angle ref"() -> (w409:dbl)
                        n3565 = local read "wavdet"() -> (w426:bool)
                        n3566 = local read "Vx-ref"() -> (w421:dbl)
                        n3567 = local read "Vy-ref"() -> (w423:dbl)
                        n3568 = local read "avpp"() -> (w422:i32)
                        n3569 = call "tt_timeandsamples.vi"("bin"=w416, "refreshtime"=w410, "srateAODOtt"=w413, "tot#ofsamples"=w418) -> ("refreshrate"=w414:dbl, "refreshbuffer"=w415:i32, "timetracecycles"=w420:i32)  [unwired: 5 in]
                        n3570 = local read "bin"() -> (w417:dbl)
                        n3571 = call "2pparameters.vi"("command"="get") -> ("params out"=w429:T10)  [unwired: 1 in]
                        n3572 = Bundle By Name(cluster=w429, "Drawing Mode"=w402, "measpoints"=w418, "tt_cycles"=w420, "refreshbuffer"=w415, "refreshrate"=w414, "Vx-ref"=w421, "Vy-ref"=w423, "srate"=w412, "finite"=w425, "cont"=w424, "wavdet"=w426, "avpp"=w422, "srateAODO"=w419, "bufferAI"=w415, "bin"=w417, "Angle Img"=w409, "Vxminref"=w408, "Vxmaxref"=w407, "Vyminref"=w406, "Vymaxref"=w405, "Xpixels Img"=w404, "Ypixels Img"=w403, "Pel"=w401, "Vz-reset"=0.0, "AIoverride"=w399, "type"="Timetrace") -> (w427:T10)
                        n3573 = Reciprocal(x=w414) -> (1/x=w411:dbl)
                        n3574 = local write "refreshtime"(w411) -> ()
                        n3575 = call "2pparameters.vi"("Params in"=w427, "command"="set") -> ()  [unwired: 1 out]
                      }
                      frame "Lifetime (point)" {
                      }
                    }
                  }
                  frame #1 {
                    w432 = FALSE ("wavdet")
                    n3576 = call "2pparameters.vi"("command"="get") -> ("params out"=w436:T10)  [unwired: 1 in]
                    n3577 = Bundle By Name(cluster=w436, "finite"=w432, "cont"=w432, "wavdet"=TRUE) -> (w433:T10)
                    n3578 = call "2pparameters.vi"("Params in"=w433, "command"="set") -> ()  [unwired: 1 out]
                  }
                  frame #2 {
                    # "remove channel from numbers array"
                    n3579 = local read "AO channels"() -> (w443:u32)
                    n3580 = call "2pparameters.vi"("command"="get") -> ("params out"=w441:T10)  [unwired: 1 in]
                    n3581 = in-place {
                      in-place-border: w443 -> [w449]
                      in-place-border: [w446] -> w444
                      in-place-border: [w445] -> w438
                      n3582 = in-place-cluster #50(w441) -> ("aAO"=w448:u32[])
                      n3583 = call "remove channel from active arrayv2.vi"("line array in"=w448, "line to remove"=w449) -> ("line array out"=w447:u32[], "removal"=w446:bool, "index"=w445:i32)
                      n3584 = in-place-cluster #50("aAO"=w447) -> (w439:T10)
                    }
                    n3585 = local write "remAO"(w444) -> ()
                    n3586 = call "2pparameters.vi"("Params in"=w439, "command"="set") -> ()  [unwired: 1 out]
                  }
                  frame #3 {
                    n3587 = local read "remAO"() -> (w450:bool)
                    n3588 = case shown="True" w450 {
                      frame False {
                      }
                      frame True {
                        n3589 = call "Used AO lines.vi"() -> ("used AO names"=w454:string[], "used AO lines"=w456:tag[])  [unwired: 2 in]
                        n3590 = control-ref of="Analog Lines Plot"() -> (w455:refnum<vi>)
                        n3591 = control-ref of="Digital Lines Plot"() -> (w453:refnum<vi>)
                        n3592 = call "Used DO lines.vi"() -> ("used DO names"=w452:string[], "used DO lines"=w451:tag[])  [unwired: 2 in]
                        n3593 = local write "Analog Used Lines"(w456) -> ()
                        n3594 = local write "Analog Used Names"(w454) -> ()
                        n3595 = local write "Digital Used Lines"(w451) -> ()
                        n3596 = local write "Digital Used Names"(w452) -> ()
                        n3597 = call "prepDOWaveplot.vi"("DigitalGraph in"=w453, "used DO names"=w452) -> ()  [unwired: 1 in]
                        n3598 = call "prepAOWaveplot.vi"("WaveformGraph in"=w455, "Analog Used Names"=w454) -> ()  [unwired: 1 in]
                      }
                    }
                  }
                  frame #4 {
                    n3599 = local read "remAO"() -> (w457:bool)
                    n3600 = case shown="True" w457 {
                      tunnel: w458 -> [_ w459]
                      frame False {
                      }
                      frame True {
                        n3601 = call "waveformparamsv2.vi"("command"="rem AO", "index"=w459) -> ()  [unwired: 3 in, 3 out]
                      }
                    }
                  }
                  frame #5 {
                    n3602 = local read "remAO"() -> (w462:bool)
                    n3603 = case shown="True" w462 {
                      tunnel: w461 -> [_ w481]
                      frame False {
                      }
                      frame True {
                        n3604 = local read "Meastab"() -> (w466:enum32{"X-Y Image", "Linescan", "Timetrace"})
                        n3605 = property on="refwf" class="Ring (strict)"() -> ("RingText.Text"=w469:string)  [unwired: 2 in, 2 out]
                        n3606 = case shown="\"Timetrace\"" w466 {
                          tunnel: [w482 w483] -> w465
                          frame "X-Y Image", Default {
                            n3607 = local read "Sampling rate"() -> (w482:dbl)
                          }
                          frame "Timetrace" {
                            n3608 = local read "srateAODOtt"() -> (w483:dbl)
                          }
                        }
                        n3609 = call "waveformsAObuffer.vi"("command"="get") -> ("AO wf out"=w478:waveform(dbl)[])  [unwired: 1 in]
                        n3610 = call "waveformsDObuffer.vi"("command"="get") -> ("DO wf out"=w475:digitalwaveform[])  [unwired: 1 in]
                        n3611 = Delete From Array(array=w478, length=1, index=w481) -> (array with subset deleted=w470:waveform(dbl)[])  [unwired: 1 out]
                        n3612 = call "correctwaveformsizetemp.vi"("new sampling frequency (Hz)"=w465, "start"=FALSE, "reference waveforms to"=w469, "Analog waveforms in"=w470, "stop"=FALSE, "Digital waveforms in"=w475) -> ("analog wf out"=w473:waveform(dbl)[], "Digital wf out"=w471:digitalwaveform[], "measpoints"=w467:i32)
                        n3613 = local write "Analog Lines Plot"(w473) -> ()
                        n3614 = call "GetNumCamFramesv2.vi"("Digital Waveform Graph"=w471) -> ("Numeric"=w472:i32)  [unwired: 10 in]
                        n3615 = local write "Digital Lines Plot"(w471) -> ()
                        n3616 = call "waveformsAObuffer.vi"("AO wf in"=w473, "command"="set") -> ()  [unwired: 1 out]
                        n3617 = call "waveformsDObuffer.vi"("DO wf in"=w471, "command"="set") -> ()  [unwired: 1 out]
                        n3618 = local read "wavdet"() -> (w468:bool)
                        n3619 = local write "Total Camera Frames"(w472) -> ()
                        n3620 = case shown="True" w468 {
                          tunnel: w467 -> [_ w484]
                          frame False {
                          }
                          frame True {
                            n3621 = local write "# of frames"(w484) -> ()
                          }
                        }
                      }
                    }
                  }
                  frame #6 {
                    w485 = FALSE ("remAO")
                    n3622 = local read "finite samples"() -> (w486:bool)
                    n3623 = local read "continuous"() -> (w487:bool)
                    n3624 = local read "wavdet"() -> (w488:bool)
                    n3625 = call "2pparameters.vi"("command"="get") -> ("params out"=w491:T10)  [unwired: 1 in]
                    n3626 = Bundle By Name(cluster=w491, "finite"=w486, "cont"=w487, "wavdet"=w488) -> (w489:T10)
                    n3627 = local write "remAO"(w485) -> ()
                    n3628 = property on="Rem AO wave" class="Bool (strict)"("Val(Sgnl)"=w485) -> ()  [unwired: 2 in, 2 out]
                    n3629 = call "2pparameters.vi"("Params in"=w489, "command"="set") -> ()  [unwired: 1 out]
                  }
                }
              }
            }
          }
          event "Add DO wave": Value Change {
            n3630 = event-data() -> ("NewVal"=w493:bool)  [unwired: 1 in, 5 out]
            n3631 = case shown="True" w493 {
              frame False {
              }
              frame True {
                n3632 = stacked-sequence {
                  seq-local: [_ _ _ _ _ w653 _ _] -> [_ _ _ _ _ _ w668 _]
                  frame #0 {
                    n3633 = local read "Measurement"() -> (w494:T4)
                    n3634 = case shown="\"X-Y-t movie\", Default" w494 {
                      frame "X-Y-t movie", Default {
                        n3635 = local read "avpp"() -> (w515:i32)
                        n3636 = local read "Angle ref"() -> (w514:dbl)
                        n3637 = local read "ROI Type"() -> (w513:u16)
                        n3638 = local read "xpixels ref"() -> (w510:i32)
                        n3639 = local read "Vx-min ref"() -> (w509:dbl)
                        n3640 = local read "Vx-max ref"() -> (w508:dbl)
                        n3641 = local read "ypixels ref"() -> (w506:i32)
                        n3642 = local read "Vy-min ref"() -> (w507:dbl)
                        n3643 = local read "Vy-max ref"() -> (w503:dbl)
                        n3644 = local read "Sampling rate"() -> (w497:dbl)
